vi "SCLC.vi"() -> ()   [LabVIEW 2015]
uses:
  SCLC_States.ctl
  <vilib>/Analysis/NI_AALPro.lvlib
panel:
  out "Transport":cluster{ext[], ext[]}[](graph)
  out "?":string
  in  "Choose File":i16 min=0 max=17
  out "Recorded Properties":T1
  out "Sample Fabrication Properties":T2
  out "DEBUG_NUMFILES":i32
  out "DEBUG_FILENAMES":string[](array[string])
  in  "stop":bool
  in  "Transport Path":path
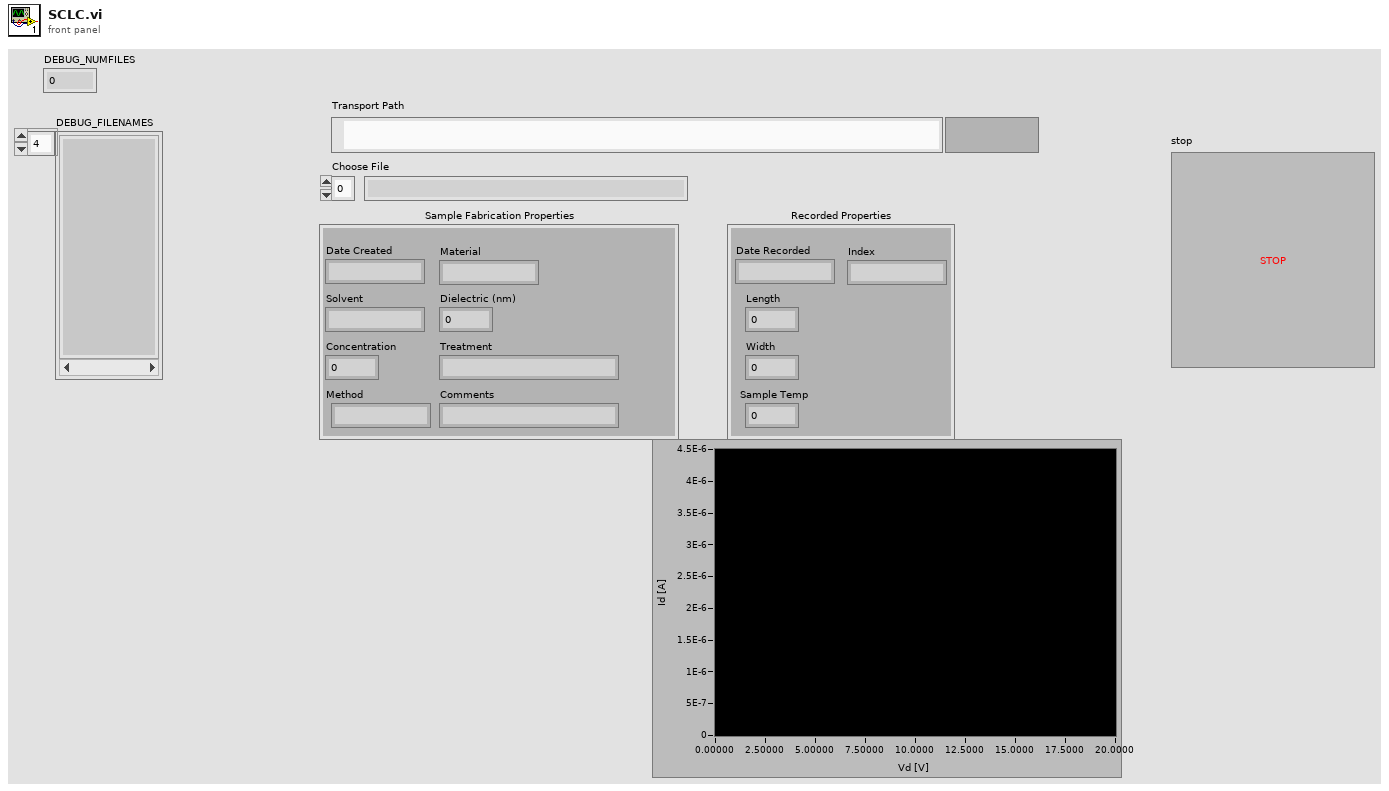
[diagram p1: front panel]
types:
  T1 = cluster{"Date Recorded":string, "Index":string, "Length":dbl, "Width":dbl, "Sample Temp":dbl}
  T2 = cluster{"Date Created":string, "Material":string, "Solvent":string, "Concentration":dbl, "Method":string, "Dielectric (nm)":dbl, "Treatment":string, "Comments":string}
  T3 = typedef "SCLC_States.ctl" = enum16{"Init", "Read", "Idle and Display", "Exit"}
  T4 = cluster{"Mobility-Sat":dbl, "Moblitity-Lin":dbl, "On/Off":dbl, "Off Current":dbl, "Vt-Sat":dbl, "STS":dbl, "Trap Density-VT":dbl, "Trap Density-STS":dbl}
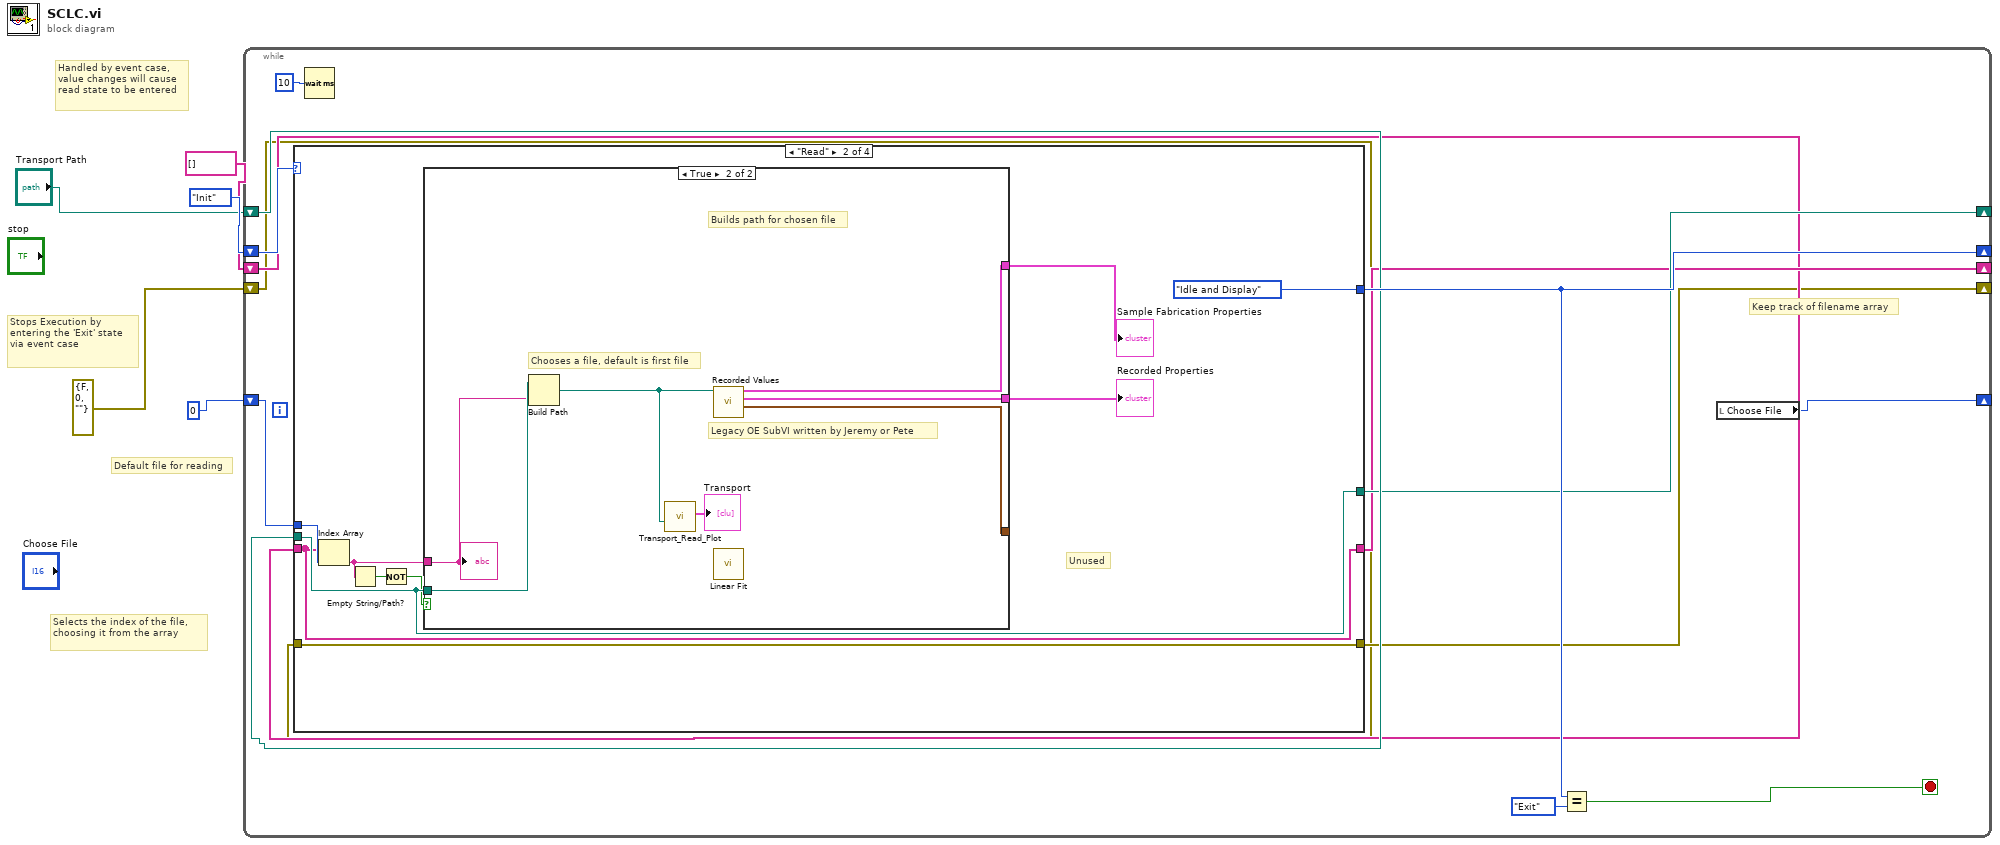
[diagram p0: block diagram]
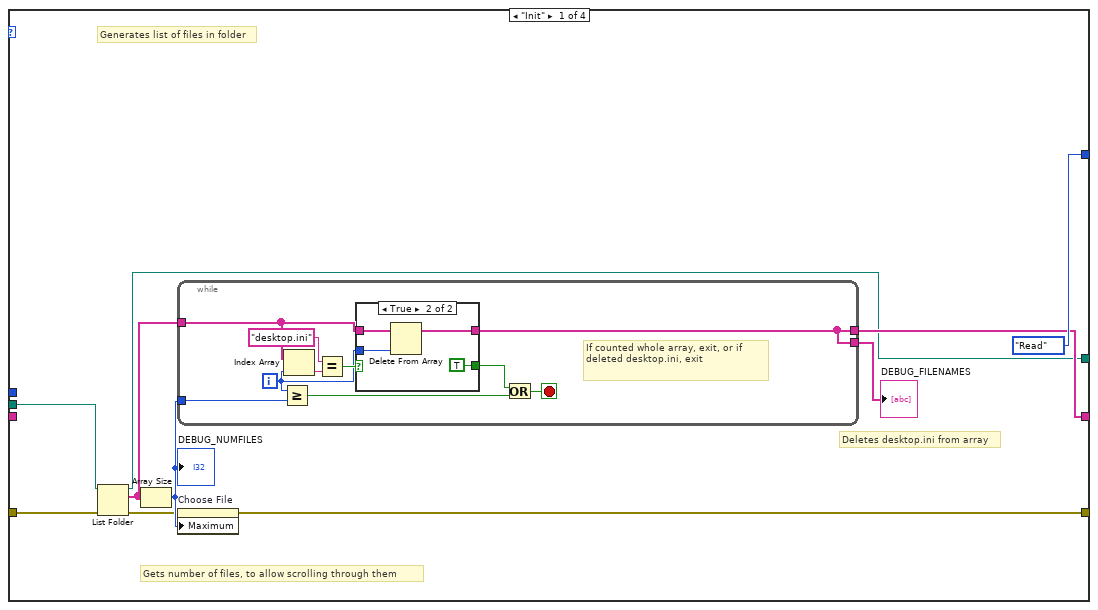
[diagram p2: hidden frame]
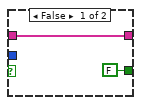
[diagram p3: hidden frame]
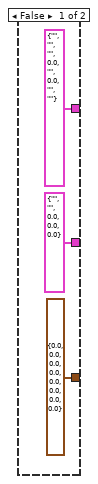
[diagram p4: hidden frame]
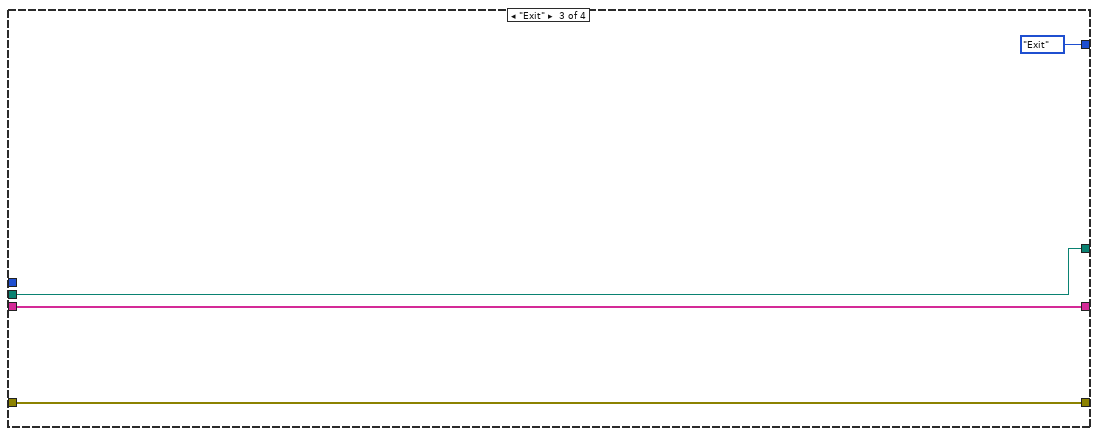
[diagram p5: hidden frame]
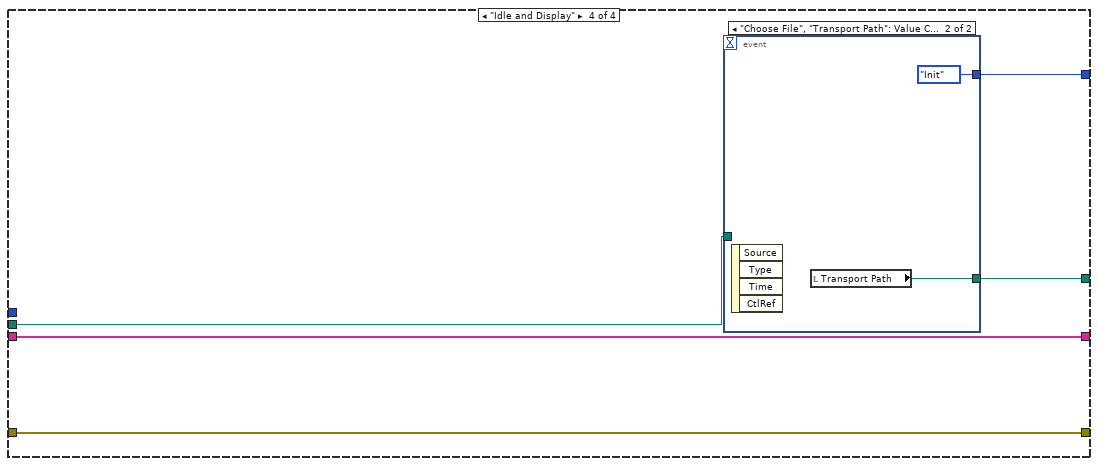
[diagram p6: hidden frame]
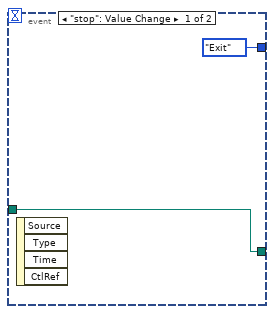
[diagram p7: hidden frame]
diagram:
  # "Selects the index of the file, choosing it from the array"
  # "Default file for reading"
  # "Handled by event case, value changes will cause read state to be entered"
  # "Stops Execution by entering the 'Exit' state via event case"
  n1 = while {
    shift-right: [w16] -> _
    shift-left: SCLC_States."Init" -> [w18]
    shift-right: [w12] -> _
    shift-left: "Transport Path" -> [w13]
    shift-right: [w11] -> _
    shift-left: string[] [] ("filenames") -> [w10]
    shift-right: [w9] -> _
    shift-left: errorcluster {"status"=FALSE, "code"=0, "source"=""} ("error in") -> [w8]
    shift-right: [w6] -> _
    shift-left: 0 -> [w7]
    stop <- w15 stop-if-true
    # "Keep track of filename array"
    n2 = case shown="\"Read\"" w18 {
      tunnel: w13 -> [w25 w52 w67 w71]
      tunnel: [SCLC_States."Read" SCLC_States."Idle and Display" SCLC_States."Exit" w73] -> w16
      tunnel: [w22 w52 w67 w72] -> w12
      tunnel: [w24 w48 w66 w70] -> w11
      tunnel: w10 -> [_ w48 w66 w70]
      tunnel: [w19 w53 w65 w69] -> w9
      tunnel: w8 -> [w23 w53 w65 w69]
      tunnel: w7 -> [_ w49 _ _]
      frame "Init" {
        # "Deletes desktop.ini from array"
        # "Gets number of files, to allow scrolling through them"
        # "Generates list of files in folder"
        n3 = List Folder(path=w25, error in=w23) -> (path out=w22:path, filenames=w27:string[], error out=w20:errorcluster)  [unwired: 2 in, 1 out]
        n4 = Array Size(array=w27) -> (size(s)=w21:i32)
        "DEBUG_NUMFILES" <- w21
        n5 = while {
          tunnel: w27 -> [w35]
          tunnel: [w30] -> w24
          tunnel: w21 -> [w34]
          tunnel: [w30] -> w26
          i -> [w29]
          stop <- w31 stop-if-true
          # "If counted whole array, exit, or if deleted desktop.ini, exit"
          n6 = Greater Or Equal?(x=w29, y=w34) -> (x >= y?=w32:bool)
          n7 = Index Array(array=w35, index=w29) -> (element=w37:string)
          n8 = Equal?(x="desktop.ini", y=w37) -> (x = y?=w36:bool)
          n9 = case shown="True" w36 {
            tunnel: w35 -> [w40 w44]
            tunnel: [w40 w43] -> w30
            tunnel: [FALSE TRUE] -> w33
            tunnel: w29 -> [_ w41]
            frame False {
            }
            frame True {
              n10 = Delete From Array(array=w44, index=w41) -> (array with subset deleted=w43:string[])  [unwired: 1 in, 1 out]
            }
          }
          n11 = Or(x=w33, y=w32) -> (x .or. y?=w31:bool)
        }
        "DEBUG_FILENAMES" <- w26
        n12 = property on="Choose File" class="DigNum (strict)"(error in=w20, "Maximum"=w21) -> (error out=w19:errorcluster)  [unwired: 1 in, 1 out]
      }
      frame "Read" {
        # "Unused"
        n13 = Index Array(array=w48, index=w49) -> (element=w47:string)
        n14 = Empty String/Path?(string/path=w47) -> (empty?=w46:bool)
        n15 = Not(x=w46) -> (.not. x?=w45:bool)
        n16 = case shown="True" w45 {
          tunnel: w52 -> [_ w60]
          tunnel: [T2 {"Date Created"="", "Material"="", "Solvent"="", "Concentration"=0.0, "Method"="", "Dielectric (nm)"=0.0, "Treatment"="", "Comments"=""} ("Fabrication Prop") w64] -> w51
          tunnel: [T1 {"Date Recorded"="", "Index"="", "Length"=0.0, "Width"=0.0, "Sample Temp"=0.0} ("Recorded Prop") w63] -> w50
          tunnel: [T4 {"Mobility-Sat"=0.0, "Moblitity-Lin"=0.0, "On/Off"=0.0, "Off Current"=0.0, "Vt-Sat"=0.0, "STS"=0.0, "Trap Density-VT"=0.0, "Trap Density-STS"=0.0} ("Recorded Char") w62] -> _
          tunnel: w47 -> [_ w59]
          frame False {
          }
          frame True {
            # "Builds path for chosen file"
            # "Chooses a file, default is first file"
            # "Legacy OE SubVI written by Jeremy or Pete"
            n17 = Build Path(base path=w60, name or relative path=w59) -> (appended path=w58:path)
            n18 = call "Transport_Read_Plot.vi"("Transport File Path"=w58) -> ("Transport"=→"Transport":cluster{ext[], ext[]}[])  [unwired: 9 in, 1 out]
            n19 = call "Recorded Values.vi"("Path"=w58) -> ("Recorded Char"=w62:T4, "Recorded Prop"=w63:T1, "Fabrication Prop"=w64:T2)  [unwired: 8 in]
            n20 = call <vilib>:"Linear Fit.vi"() -> ()  [unwired: 11 in, 5 out]
            "?" <- w59
          }
        }
        "Sample Fabrication Properties" <- w51
        "Recorded Properties" <- w50
      }
      frame "Exit" {
      }
      frame "Idle and Display" {
        n21 = event shown="[1] \"Choose File\", \"Transport Path\": Value Change" {
          selector: _ -> [_ _]
          dyn-events: _ -> [_ _]
          timeout: _ -> [_ _]
          tunnel: [SCLC_States."Exit" SCLC_States."Init"] -> w73
          tunnel: [w74 w77] -> w72
          tunnel: w71 -> [w74 _]
          event "stop": Value Change {
            n22 = event-data() -> ()  [unwired: 1 in, 4 out]
          }
          event "Choose File", "Transport Path": Value Change {
            n23 = event-data() -> ()  [unwired: 1 in, 4 out]
            n24 = local read "Transport Path"() -> (w77:path)
          }
        }
      }
    }
    n25 = Wait (ms)(milliseconds to wait=u32 10) -> ()  [unwired: 1 out]
    n26 = Equal?(x=w16, y=SCLC_States."Exit") -> (x = y?=w15:bool)
    n27 = local read "Choose File"() -> (w6:i16)
  }
